vi "Get next state for the run loop.vi"(0 "Loop order":T1, 1 "Last setting":bool, 2 "Last Power?":bool, 3 "Last Frequency?":bool, 4 "Last Offset?":bool, 7 "Last Power Delta?":bool) -> (14 "Run states":T2)   [LabVIEW 2020, in "IMD.lvclass"]
uses:
  IMD.lvclass
  Controls/Run states.ctl
  Controls/Loop order.ctl
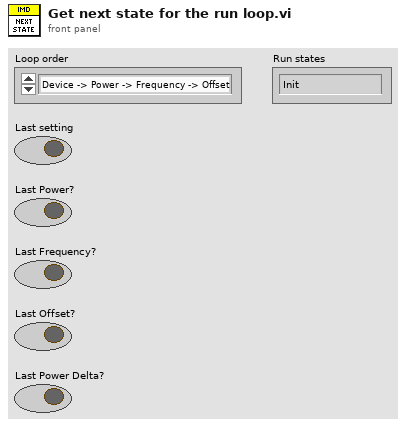
[diagram p1: front panel]
types:
  T1 = typedef "IMD.lvclass/Loop order.ctl" = enum16{"Device -> Power -> Frequency -> Offset", "Device -> Frequency -> Power -> Offset"}
  T2 = typedef "IMD.lvclass/Run states.ctl" = enum16{"Init", "Set Device", "Set Power", "Set Delta Power", "Set Frequency", "Set Offset", "Measure", "Done"}
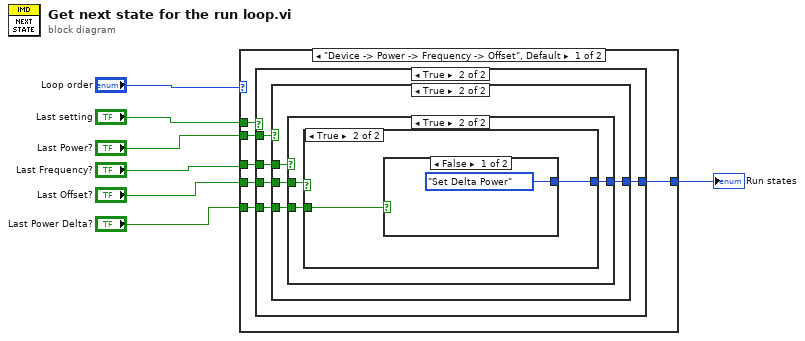
[diagram p0: block diagram]
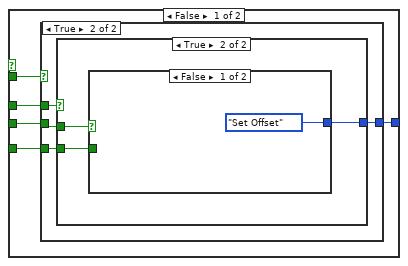
[diagram p2: hidden frame]
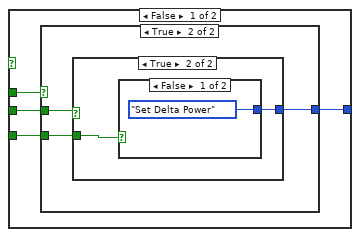
[diagram p3: hidden frame]
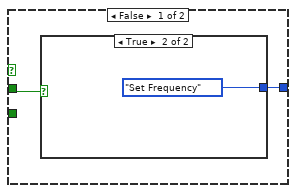
[diagram p4: hidden frame]
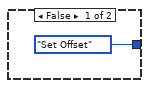
[diagram p5: hidden frame]
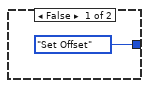
[diagram p6: hidden frame]
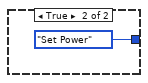
[diagram p7: hidden frame]
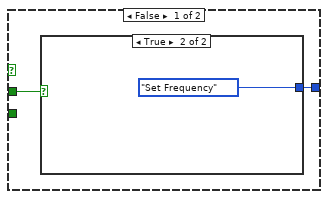
[diagram p8: hidden frame]
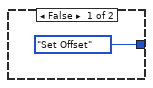
[diagram p9: hidden frame]
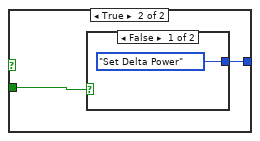
[diagram p10: hidden frame]
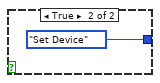
[diagram p11: hidden frame]
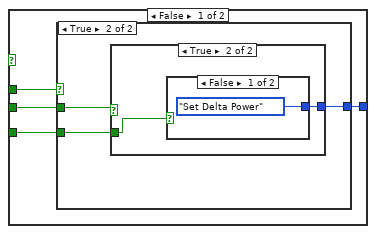
[diagram p12: hidden frame]
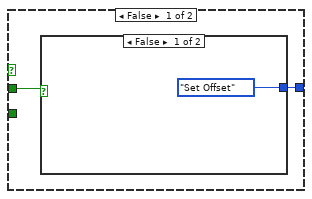
[diagram p13: hidden frame]
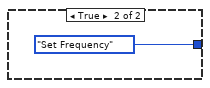
[diagram p14: hidden frame]
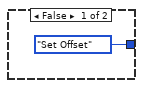
[diagram p15: hidden frame]
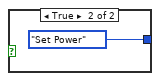
[diagram p16: hidden frame]
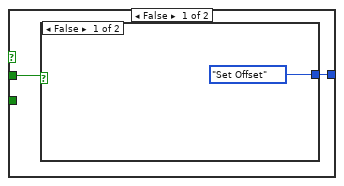
[diagram p17: hidden frame]
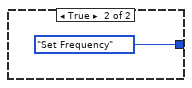
[diagram p18: hidden frame]
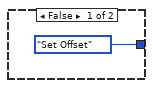
[diagram p19: hidden frame]
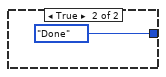
[diagram p20: hidden frame]
diagram:
  n1 = case shown="\"Device -> Power -> Frequency -> Offset\", Default" "Loop order" {
    tunnel: "Last setting" -> [w13 w93]
    tunnel: "Last Power?" -> [w12 w92]
    tunnel: "Last Frequency?" -> [w11 w91]
    tunnel: [w10 w90] -> w7
    tunnel: "Last Offset?" -> [w9 w89]
    tunnel: "Last Power Delta?" -> [w8 w88]
    frame "Device -> Power -> Frequency -> Offset", Default {
      n2 = case shown="True" w13 {
        tunnel: w12 -> [w18 w55]
        tunnel: w11 -> [w17 w54]
        tunnel: [w16 w53] -> w10
        tunnel: w9 -> [w15 w52]
        tunnel: w8 -> [w14 w51]
        frame False {
          n3 = case shown="True" w18 {
            tunnel: w17 -> [w22 w38]
            tunnel: [w21 w37] -> w16
            tunnel: w15 -> [w20 w36]
            tunnel: w14 -> [w19 w35]
            frame False {
              n4 = case shown="True" w22 {
                tunnel: [w24 w29] -> w21
                tunnel: w20 -> [w23 w28]
                tunnel: w19 -> [_ w27]
                frame False {
                  n5 = case shown="True" w23 {
                    tunnel: [Run_states."Set Offset" ("Run states") Run_states."Set Frequency" ("Run states")] -> w24
                    frame False {
                    }
                    frame True {
                    }
                  }
                }
                frame True {
                  n6 = case shown="True" w28 {
                    tunnel: [Run_states."Set Offset" ("Run states") w32] -> w29
                    tunnel: w27 -> [_ w31]
                    frame False {
                    }
                    frame True {
                      n7 = case shown="False" w31 {
                        tunnel: [Run_states."Set Delta Power" ("Run states") Run_states."Set Power" ("Run states")] -> w32
                        frame False {
                        }
                        frame True {
                        }
                      }
                    }
                  }
                }
              }
            }
            frame True {
              n8 = case shown="True" w38 {
                tunnel: [w40 w45] -> w37
                tunnel: w36 -> [w39 w44]
                tunnel: w35 -> [_ w43]
                frame False {
                  n9 = case shown="True" w39 {
                    tunnel: [Run_states."Set Offset" ("Run states") Run_states."Set Frequency" ("Run states")] -> w40
                    frame False {
                    }
                    frame True {
                    }
                  }
                }
                frame True {
                  n10 = case shown="False" w44 {
                    tunnel: [Run_states."Set Offset" ("Run states") w48] -> w45
                    tunnel: w43 -> [_ w47]
                    frame False {
                    }
                    frame True {
                      n11 = case shown="False" w47 {
                        tunnel: [Run_states."Set Delta Power" ("Run states") Run_states."Set Device" ("Run states")] -> w48
                        frame False {
                        }
                        frame True {
                        }
                      }
                    }
                  }
                }
              }
            }
          }
        }
        frame True {
          n12 = case shown="True" w55 {
            tunnel: w54 -> [w59 w75]
            tunnel: [w58 w74] -> w53
            tunnel: w52 -> [w57 w73]
            tunnel: w51 -> [w56 w72]
            frame False {
              n13 = case shown="True" w59 {
                tunnel: [w61 w66] -> w58
                tunnel: w57 -> [w60 w65]
                tunnel: w56 -> [_ w64]
                frame False {
                  n14 = case shown="False" w60 {
                    tunnel: [Run_states."Set Offset" ("Run states") Run_states."Set Frequency" ("Run states")] -> w61
                    frame False {
                    }
                    frame True {
                    }
                  }
                }
                frame True {
                  n15 = case shown="True" w65 {
                    tunnel: [Run_states."Set Offset" ("Run states") w69] -> w66
                    tunnel: w64 -> [_ w68]
                    frame False {
                    }
                    frame True {
                      n16 = case shown="False" w68 {
                        tunnel: [Run_states."Set Delta Power" ("Run states") Run_states."Set Power" ("Run states")] -> w69
                        frame False {
                        }
                        frame True {
                        }
                      }
                    }
                  }
                }
              }
            }
            frame True {
              n17 = case shown="True" w75 {
                tunnel: [w77 w82] -> w74
                tunnel: w73 -> [w76 w81]
                tunnel: w72 -> [_ w80]
                frame False {
                  n18 = case shown="False" w76 {
                    tunnel: [Run_states."Set Offset" ("Run states") Run_states."Set Frequency" ("Run states")] -> w77
                    frame False {
                    }
                    frame True {
                    }
                  }
                }
                frame True {
                  n19 = case shown="True" w81 {
                    tunnel: [Run_states."Set Offset" ("Run states") w85] -> w82
                    tunnel: w80 -> [_ w84]
                    frame False {
                    }
                    frame True {
                      n20 = case shown="False" w84 {
                        tunnel: [Run_states."Set Delta Power" ("Run states") Run_states."Done" ("Run states")] -> w85
                        frame False {
                        }
                        frame True {
                        }
                      }
                    }
                  }
                }
              }
            }
          }
        }
      }
    }
    frame "Device -> Frequency -> Power -> Offset" {
      n21 = case shown="False" w93 {
        tunnel: w92 -> [w98 w127]
        tunnel: w91 -> [w97 w126]
        tunnel: [w96 w125] -> w90
        tunnel: w89 -> [w95 w124]
        tunnel: w88 -> [w94 w123]
        frame False {
          n22 = case shown="True" w98 {
            tunnel: w97 -> [_ w110]
            tunnel: [w101 w109] -> w96
            tunnel: w95 -> [w100 w108]
            tunnel: w94 -> [w99 w107]
            frame False {
              n23 = case shown="True" w100 {
                tunnel: [Run_states."Set Offset" ("Run states") w104] -> w101
                tunnel: w99 -> [_ w103]
                frame False {
                }
                frame True {
                  n24 = case shown="False" w103 {
                    tunnel: [Run_states."Set Delta Power" ("Run states") Run_states."Set Power" ("Run states")] -> w104
                    frame False {
                    }
                    frame True {
                    }
                  }
                }
              }
            }
            frame True {
              n25 = case shown="True" w110 {
                tunnel: [w112 w117] -> w109
                tunnel: w108 -> [w111 w116]
                tunnel: w107 -> [_ w115]
                frame False {
                  n26 = case shown="False" w111 {
                    tunnel: [Run_states."Set Offset" ("Run states") Run_states."Set Frequency" ("Run states")] -> w112
                    frame False {
                    }
                    frame True {
                    }
                  }
                }
                frame True {
                  n27 = case shown="False" w116 {
                    tunnel: [Run_states."Set Offset" ("Run states") w120] -> w117
                    tunnel: w115 -> [_ w119]
                    frame False {
                    }
                    frame True {
                      n28 = case shown="False" w119 {
                        tunnel: [Run_states."Set Delta Power" ("Run states") Run_states."Set Device" ("Run states")] -> w120
                        frame False {
                        }
                        frame True {
                        }
                      }
                    }
                  }
                }
              }
            }
          }
        }
        frame True {
          n29 = case shown="True" w127 {
            tunnel: w126 -> [w131 _]
            tunnel: [w130 w150] -> w125
            tunnel: w124 -> [w129 w149]
            tunnel: w123 -> [w128 w148]
            frame True {
              n30 = case shown="False" w131 {
                tunnel: [w134 w142] -> w130
                tunnel: w129 -> [w133 w141]
                tunnel: w128 -> [w132 w140]
                frame False {
                  n31 = case shown="True" w133 {
                    tunnel: [Run_states."Set Offset" ("Run states") w137] -> w134
                    tunnel: w132 -> [_ w136]
                    frame False {
                    }
                    frame True {
                      n32 = case shown="True" w136 {
                        tunnel: [Run_states."Set Delta Power" ("Run states") Run_states."Set Frequency" ("Run states")] -> w137
                        frame False {
                        }
                        frame True {
                        }
                      }
                    }
                  }
                }
                frame True {
                  n33 = case shown="True" w141 {
                    tunnel: [Run_states."Set Offset" ("Run states") w145] -> w142
                    tunnel: w140 -> [_ w144]
                    frame False {
                    }
                    frame True {
                      n34 = case shown="False" w144 {
                        tunnel: [Run_states."Set Delta Power" ("Run states") Run_states."Done" ("Run states")] -> w145
                        frame False {
                        }
                        frame True {
                        }
                      }
                    }
                  }
                }
              }
            }
            frame False {
              n35 = case shown="True" w149 {
                tunnel: [Run_states."Set Offset" ("Run states") w153] -> w150
                tunnel: w148 -> [_ w152]
                frame False {
                }
                frame True {
                  n36 = case shown="False" w152 {
                    tunnel: [Run_states."Set Delta Power" ("Run states") Run_states."Set Power" ("Run states")] -> w153
                    frame False {
                    }
                    frame True {
                    }
                  }
                }
              }
            }
          }
        }
      }
    }
  }
  "Run states" <- w7
